vi "Harry_kane_1.0.vi"() -> ()   [LabVIEW 2013]
uses:
  <vilib>/vision/NI_Vision_Development_Module.lvlib
panel:
  in  "Calibrate":bool
  in  "File Path (Image Calibration 1)":path=path "\\\\hs2.lboro.ac.uk\\mmbc4/1_Univesity Work/Mechatronics/Machine Vision/Harry_Kane_Project/A3_table_cal_2.png"
  out "Y Co-ordinate (pixels)":dbl[](array[numeric])
  out "X Co ordinate (pixels)":dbl[](array[numeric])
  out "Reference Point in pixels\n (intersection)":cluster{"X":sgl, "Y":sgl} {"Y" format="%.2f"; "X" format="%.2f"}
  out "Circles Data (Circle Detection 1)":T1(array[cluster])
  out "Particle Measurements (Pixels) (Circle Analysis)":dbl[][](array[numeric]) format="%.2f"
  out "Image in":T2(plugin-control)
  in  "Stop":bool
  out "Binary":T2(plugin-control)
  in  "Capture image":bool
  out "Calibrated":T2(plugin-control)
  in  "File Path":path
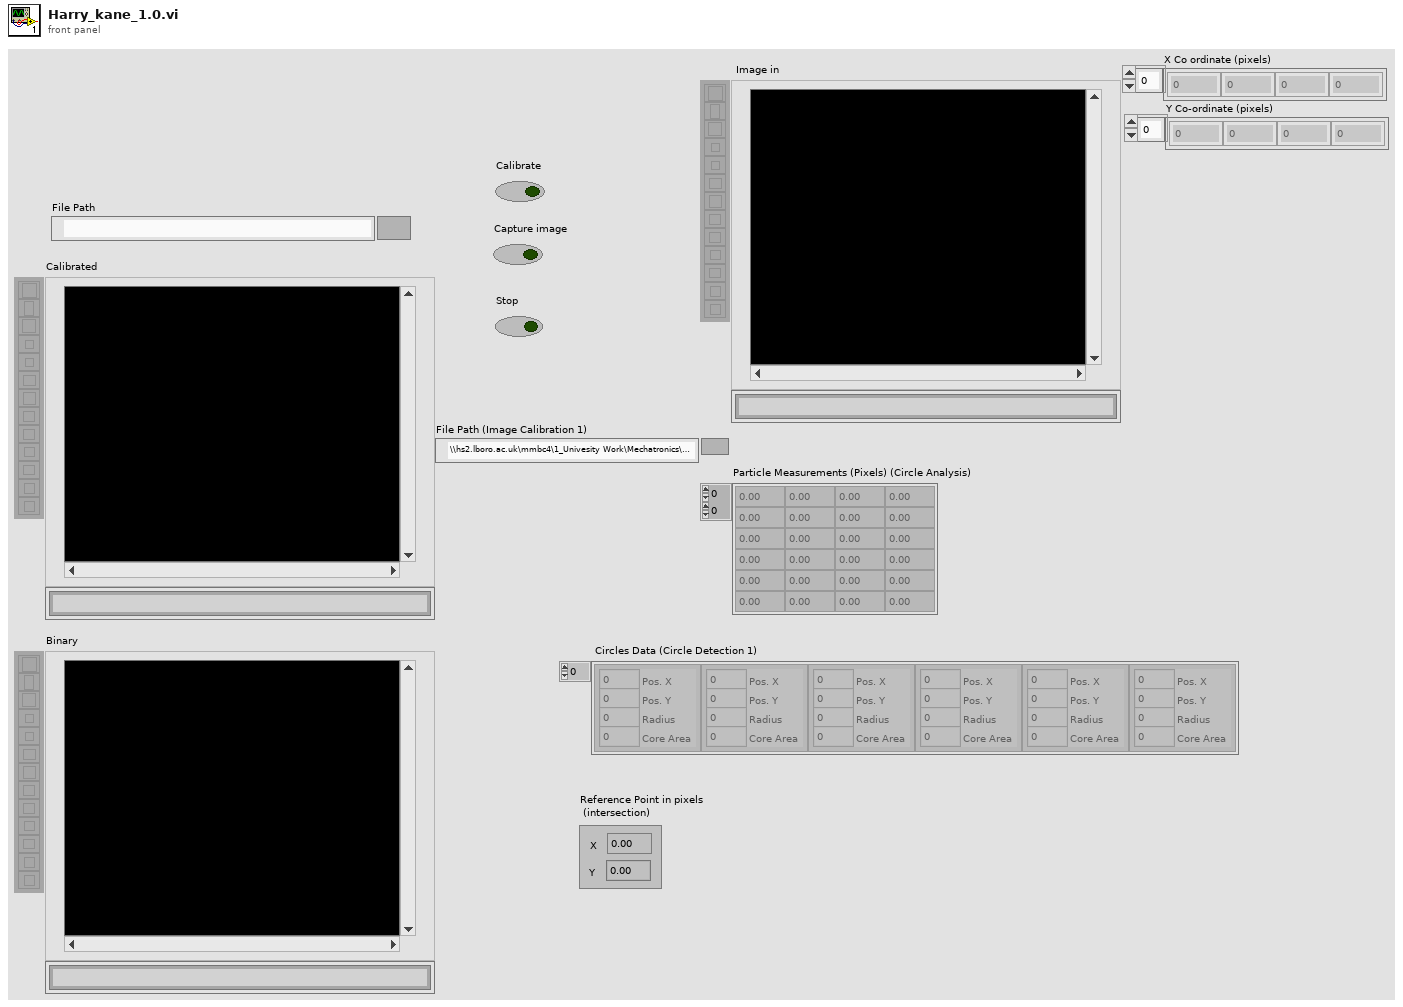
[diagram p1: front panel]
types:
  T1 = cluster{"Pos. X":i32, "Pos. Y":i32, "Radius":i32, "Core Area":i32}[]
  T2 = typedef "IMAQ Image.ctl" = refnum<image>
  T3 = typedef "Image Type" = u32
  T4 = cluster{"Point1 (Pixels)":cluster{"X":sgl, "Y":sgl}, "Point2 (Pixels)":cluster{"X":sgl, "Y":sgl}, "Point1 (Real-World)":cluster{"X":sgl, "Y":sgl}, "Point2 (Real-World)":cluster{"X":sgl, "Y":sgl}, "Angle (Pixel)":dbl, "Angle (Real-World)":dbl, "Score":dbl, "Straightness":dbl, "Average SNR (db)":dbl, "Calibration Valid":bool}
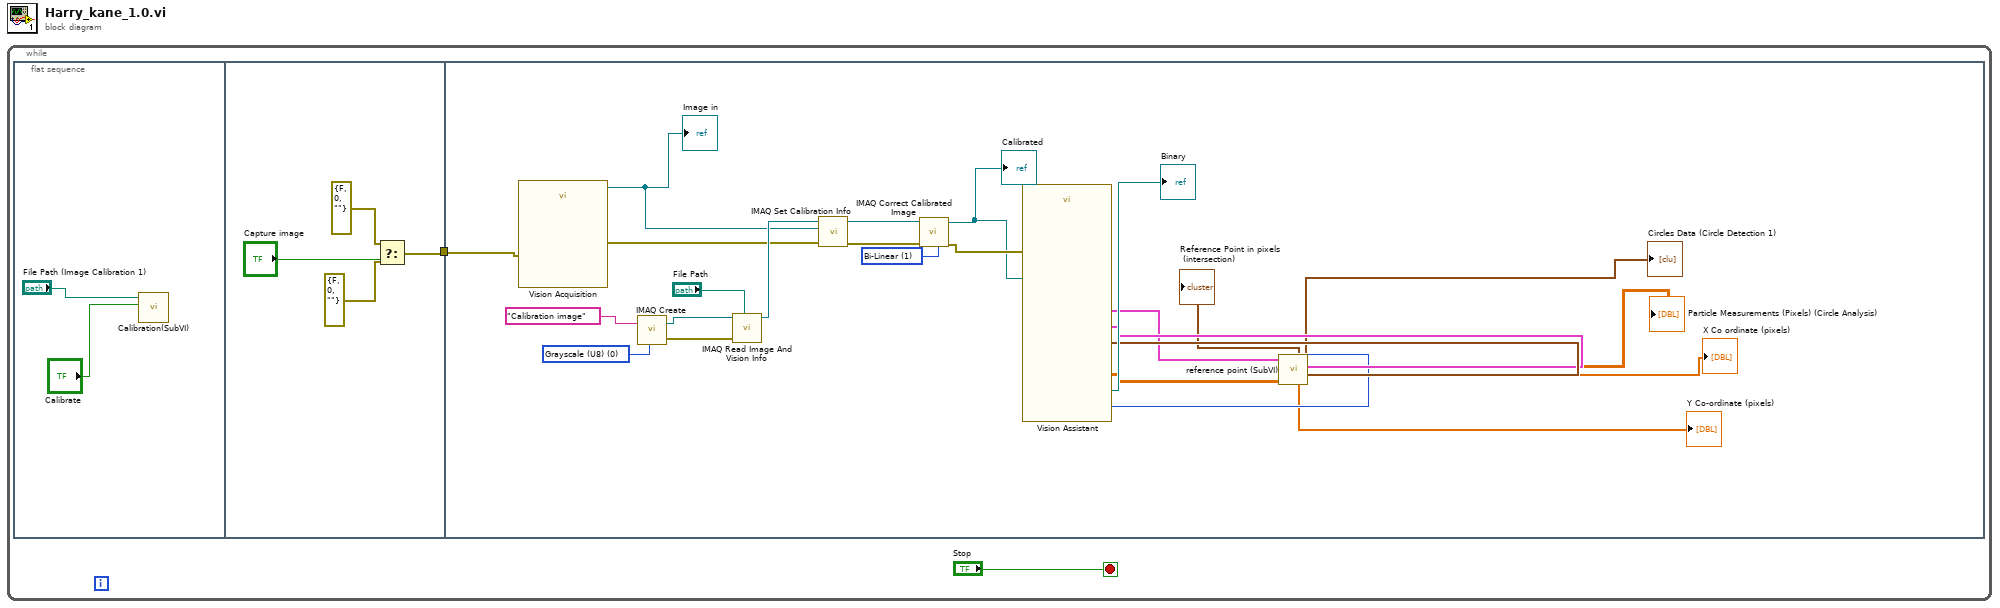
[diagram p0: block diagram]
diagram:
  n1 = while {
    stop <- "Stop" stop-if-true
    n2 = flat-sequence {
      tunnel: [w5] -> w1
      tunnel: w1 -> [w21]
      frame #0 {
        n3 = call "Calibration(SubVI).vi"("Calibrate"="Calibrate", "File Path (Image Calibration 1)"="File Path (Image Calibration 1)") -> ()  [unwired: 8 in, 2 out]
      }
      frame #1 {
        n4 = Select(t=errorcluster {"status"=FALSE, "code"=0, "source"=""} ("error in"), s="Capture image", f=errorcluster {"status"=FALSE, "code"=0, "source"=""} ("error in")) -> (s? t:f=w5:errorcluster)
      }
      frame #2 {
        w28 = T3 0 items=["Grayscale (U8)", "Grayscale (I16)", "Grayscale (SGL)", "Complex (CSG)", "RGB (U32)", "HSL (U32)", "RGB (U64)", "Grayscale (U16)"] ("Image Type")
        w27 = u32 1 items=["Zero Order", "Bi-Linear", "Quadratic", "Cubic Spline"] ("Interpolation Type")
        n5 = call "Vision Acquisition"("error in"=w21) -> ("Image Out"=w23:T2, "error out"=w22:errorcluster)  [unwired: 25 in]
        "Image in" <- w23
        n6 = call "IMAQ Create"("Image Name"="Calibration image", "Image Type"=w28) -> ("New Image"=w33:T2, "error out"=w32:errorcluster)  [unwired: 3 in]
        n7 = call "IMAQ Read Image And Vision Info"("File Path"="File Path", "error in (no error)"=w32, "Image"=w33) -> ("Image Out"=w31:T2)  [unwired: 6 in, 2 out]
        n8 = call "IMAQ Set Calibration Info"("error in (no error)"=w22, "Image Dst"=w23, "Image Src"=w31) -> ("error out"=w26:errorcluster, "Calibrated Image"=w30:T2)  [unwired: 7 in]
        n9 = call "IMAQ Correct Calibrated Image"("Interpolation Type"=w27, "error in (no error)"=w26, "Image Src"=w30) -> ("error out"=w25:errorcluster, "Corrected Image"=w18:T2)  [unwired: 7 in]
        "Calibrated" <- w18
        n10 = call "Vision Assistant"("Image In"=w18, "error in"=w25) -> ("Image Out"=→"Binary":T2, "Particle Measurements (Pixels) (Circle Analysis)"=w15:dbl[][], "Circles Data (Circle Detection 1)"=w20:T1, "Straight Edge (Find Straight Edge 1)"=w16:T4, "Straight Edge (Find Straight Edge 2)"=w17:T4, "Nb Circles (Circle Detection 1)"=w14:i32)  [unwired: 18 in, 2 out]
        n11 = call "reference point (SubVI).vi"("Particle Measurements (Pixels) (Circle Analysis) in"=w15, "Nb Circles (Circle Detection 1)"=w14, "Circles Data (Circle Detection 1) in"=w20, "Straight Edge (Find Straight Edge 2)"=w17, "Straight Edge (Find Straight Edge 1)"=w16) -> ("X Co ordinate (pixels)"=→"X Co ordinate (pixels)":dbl[], "Particle Measurements (Pixels) (Circle Analysis) out"=→"Particle Measurements (Pixels) (Circle Analysis)":dbl[][], "Circles Data (Circle Detection 1) out"=→"Circles Data (Circle Detection 1)":T1, "Y Co-ordinate (pixels)"=→"Y Co-ordinate (pixels)":dbl[], "Reference Point in pixels\n (intersection)"=→"Reference Point in pixels\n (intersection)":cluster{"X":sgl, "Y":sgl})  [unwired: 2 in]
      }
    }
  }
